vi "parse.clz.characters.vi"(1 "characters string":string) -> (0 "character":T1)   [LabVIEW 2024]
uses:
  <vilib>/Utility/error.llb/Trim Whitespace One-Sided.vi
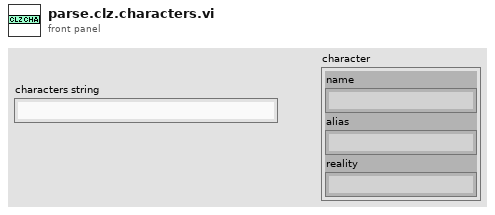
[diagram p1: front panel]
types:
  T1 = cluster{"name":string, "alias":string, "reality":string}
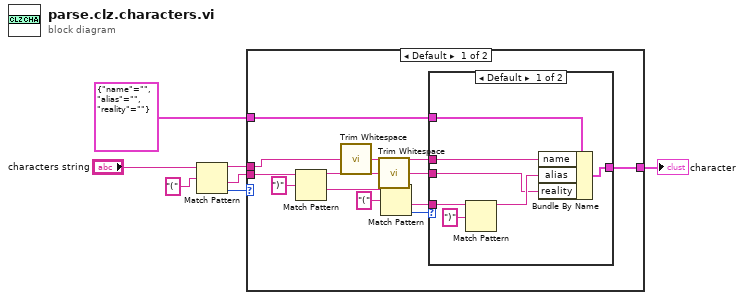
[diagram p0: block diagram]
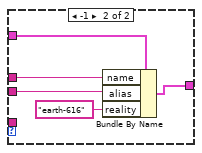
[diagram p2: hidden frame]
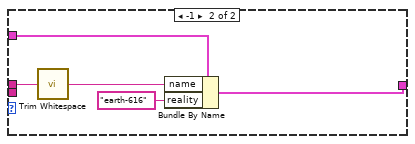
[diagram p3: hidden frame]
diagram:
  n1 = Match Pattern(string="characters string", regular expression="(") -> (before substring=w6:string, after substring=w3:string, offset past match=w5:i32)  [unwired: 1 in, 1 out]
  n2 = case shown="Default" w5 {
    tunnel: w6 -> [w17 w36]
    tunnel: w3 -> [w19 _]
    tunnel: [w10 w33] -> w1
    tunnel: T1 {"name"="", "alias"="", "reality"=""} -> [w8 w35]
    frame Default {
      n3 = Match Pattern(string=w19, regular expression=")") -> (before substring=w16:string, after substring=w15:string)  [unwired: 1 in, 2 out]
      n4 = call <vilib>:"Trim Whitespace.vi"("string"=w17) -> ("trimmed string"=w12:string)  [unwired: 1 in]
      n5 = call <vilib>:"Trim Whitespace.vi"("string"=w16) -> ("trimmed string"=w11:string)  [unwired: 1 in]
      n6 = Match Pattern(string=w15, regular expression="(") -> (after substring=w9:string, offset past match=w13:i32)  [unwired: 1 in, 2 out]
      n7 = case shown="Default" w13 {
        tunnel: w12 -> [w23 w30]
        tunnel: w11 -> [w21 w29]
        tunnel: [w20 w27] -> w10
        tunnel: w9 -> [w26 _]
        tunnel: w8 -> [w24 w31]
        frame Default {
          n8 = Match Pattern(string=w26, regular expression=")") -> (before substring=w22:string)  [unwired: 1 in, 3 out]
          n9 = Bundle By Name(cluster=w24, "name"=w23, "alias"=w22, "reality"=w21) -> (w20:T1)
        }
        frame -1 {
          n10 = Bundle By Name(cluster=w31, "name"=w30, "alias"=w29, "reality"="earth-616") -> (w27:T1)
        }
      }
    }
    frame -1 {
      n11 = call <vilib>:"Trim Whitespace.vi"("string"=w36) -> ("trimmed string"=w34:string)  [unwired: 1 in]
      n12 = Bundle By Name(cluster=w35, "name"=w34, "reality"="earth-616") -> (w33:T1)
    }
  }
  "character" <- w1
